vi "Add WAMP-CRA authenticator.vi"(7 "PBKDF2 hash type":T1, 8 "error in (no error)":errorcluster, 9 "Secret":string, 10 "Authentication ID":string, 11 "WAMP Client in":refnum<class "WAMP Client.lvclass">) -> (0 "error out":errorcluster, 3 "WAMP Client out":refnum<class "WAMP Client.lvclass">)   [LabVIEW 2020, in "wamplv.lvlib" / "WAMP Client.lvclass"]
uses:
  WAMP Client.lvclass
  Private/PBKDF2 serialisation method.ctl
  Private/Authenticators/WampCraAuthenticator/WampCraAuthenticator.lvclass
  C:/local/wamplv/Private/Authenticators/IAuthenticator/IAuthenticator.lvclass
  WAMP Client.lvclass/WAMP Client.ctl
  wamplv.lvlib
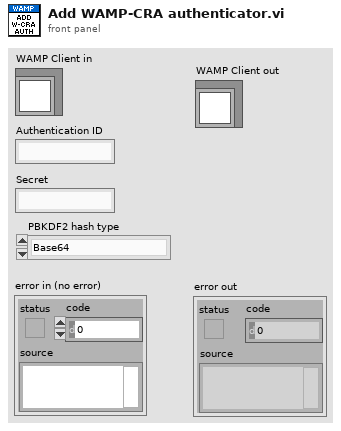
[diagram p1: front panel]
types:
  T1 = typedef "wamplv.lvlib/PBKDF2 serialisation method.ctl" = enum8{"Base64", "Hex string, lower case", "Hex string, upper case", "Direct to string cast"}
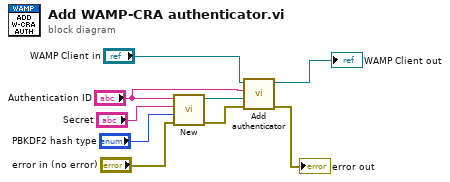
[diagram p0: block diagram]
diagram:
  n1 = call "New.vi"("error in (no error)"="error in (no error)", "PBKDF2 hash type"="PBKDF2 hash type", "Secret"="Secret", "Auth ID"="Authentication ID") -> ("error out"=w4:errorcluster, "output cluster"=w7:refnum<class "WampCraAuthenticator.lvclass">)  [unwired: 6 in]
  n2 = call "Add authenticator.vi"("error in (no error)"=w4, "IAuthenticator"=w7, "Authentication ID"="Authentication ID", "WAMP Client in"="WAMP Client in") -> ("error out"=→"error out":errorcluster, "WAMP Client out"=→"WAMP Client out":refnum<class "WAMP Client.lvclass">)  [unwired: 6 in]
